vi "Stop Lighting Effects.vi"(8 "error in (no error)":errorcluster) -> (0 "error out":errorcluster)   [LabVIEW 2025, in "Logitech Devices.lvlib"]
uses:
  Logitech Devices.lvlib
  <vilib>/Utility/error.llb/Error Cluster From Error Code.vi
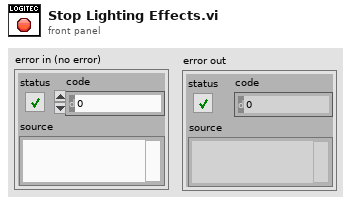
[diagram p1: front panel]
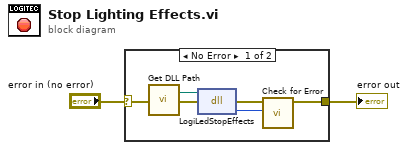
[diagram p0: block diagram]
diagram:
  n1 = case shown="No Error" "error in (no error)" {
    selector: "error in (no error)" -> [w7 w8]
    tunnel: [w4 w8] -> w1
    frame No Error {
      n2 = call "Get DLL Path.vi"() -> ("LG Hub SDK DLL"=w3:path)  [unwired: 3 in]
      n3 = dll-call lib="C:/Program Files/LGHUB/sdks/sdk_legacy_led_x86.dll" fn="LogiLedStopEffects"(path in=w3, error in=w7) -> (error out=w5:errorcluster, "return type"=w6:u8)  [unwired: 1 in, 1 out]
      n4 = call "Check for Error.vi"("DLL-call return value"=w6, "error in (no error)"=w5) -> ("error out"=w4:errorcluster)  [unwired: 9 in]
    }
    frame Error {
    }
  }
  "error out" <- w1
